vi "Enqueue Message (Single).vi"(6 "High Priority?":bool, 8 "error in (no error)":errorcluster, 9 "Data":variant, 10 "State":string, 11 "Message Queue in":refnum<queue>) -> (0 "error out":errorcluster, 3 "Message Queue out":refnum<queue>)   [LabVIEW 2016, in "Message Queue.lvlib"]
uses:
  Message Queue.lvlib
  Message.ctl
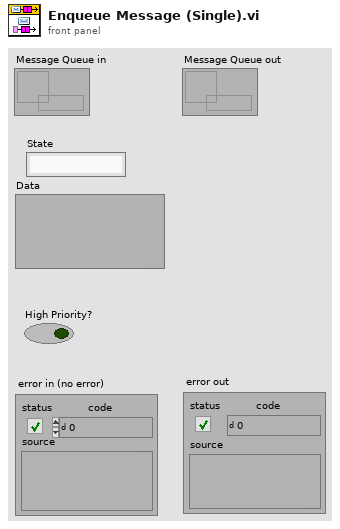
[diagram p1: front panel]
types:
  T1 = typedef "Message Queue.lvlib/Message.ctl" = cluster{"State":string, "Data":variant}
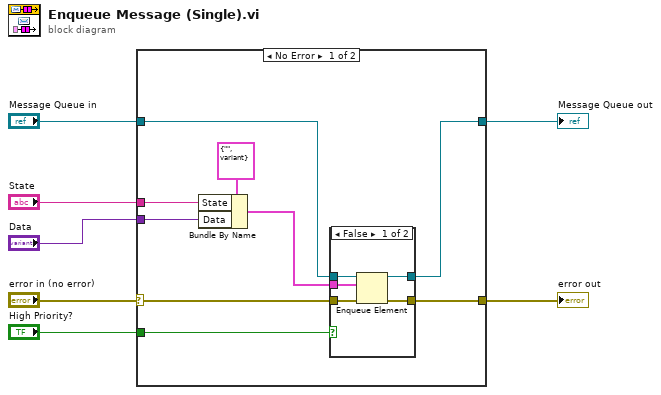
[diagram p0: block diagram]
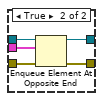
[diagram p2: hidden frame]
diagram:
  n1 = case shown="No Error" "error in (no error)" {
    selector: "error in (no error)" -> [w13 w28]
    tunnel: [w12 w28] -> w6
    tunnel: "State" -> [w15 _]
    tunnel: "Data" -> [w14 _]
    tunnel: "Message Queue in" -> [w10 w27]
    tunnel: [w9 w27] -> w2
    tunnel: "High Priority?" -> [w8 _]
    frame No Error {
      n2 = Bundle By Name(cluster=T1 {"State"="", "Data"=variant} ("Message"), "State"=w15, "Data"=w14) -> (w11:T1)
      n3 = case shown="False" w8 {
        tunnel: w13 -> [w21 w26]
        tunnel: [w20 w25] -> w12
        tunnel: w11 -> [w17 w22]
        tunnel: w10 -> [w19 w24]
        tunnel: [w18 w23] -> w9
        frame False {
          n4 = Enqueue Element(queue=w19, element=w17, error in (no error)=w21) -> (queue out=w18:refnum<queue>, error out=w20:errorcluster)  [unwired: 1 in, 1 out]
        }
        frame True {
          n5 = Enqueue Element At Opposite End(queue=w24, element=w22, error in (no error)=w26) -> (queue out=w23:refnum<queue>, error out=w25:errorcluster)  [unwired: 1 in, 1 out]
        }
      }
    }
    frame Error {
    }
  }
  "error out" <- w6
  "Message Queue out" <- w2
